vi "Max_Min_Delta.vi"() -> ()   [LabVIEW 2014]
panel:
  in  "OK Button 2":bool
  out "Delta":dbl
  out "Min":dbl
  out "Max":dbl
  in  "OK Button":bool
  in  "stop":bool
  out "Waveform Chart":dbl(graph)
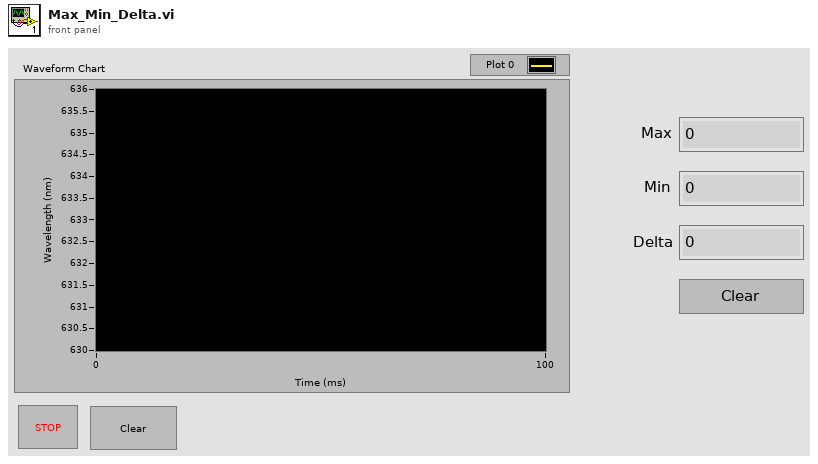
[diagram p1: front panel]
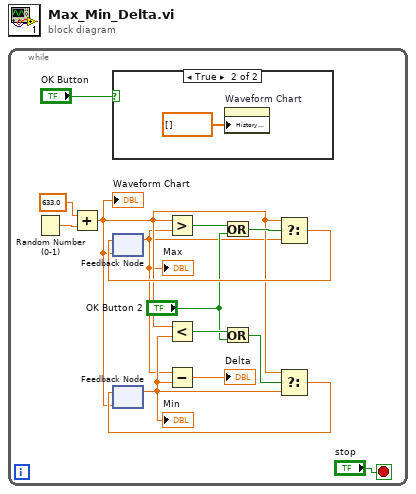
[diagram p0: block diagram]
diagram:
  n1 = while {
    stop <- "stop" stop-if-true
    n2 = Random Number (0-1)() -> (number: 0 to 1=w13:dbl)
    n3 = Add(x=633.0, y=w13) -> (x+y=w4:dbl)
    "Waveform Chart" <- w4
    n4 = case shown="True" "OK Button" {
      frame False {
      }
      frame True {
        n5 = property on="Waveform Chart" class="WFChart (strict)"("History Data"=dbl[] []) -> ()  [unwired: 2 in, 2 out]
      }
    }
    n6 = feedback #1(w4) -> (w1:dbl)
    "Max" <- w1
    n7 = feedback #2(w4) -> (w2:dbl)
    "Min" <- w2
    n8 = Greater?(x=w4, y=w1) -> (0:w11:bool)
    n9 = Less?(x=w4, y=w2) -> (x < y?=w8:bool)
    n10 = Subtract(x=w1, y=w2) -> (x-y=→"Delta":dbl)
    n11 = Or(x=w11, y="OK Button 2") -> (x .or. y?=w10:bool)
    n12 = Or(x=w8, y="OK Button 2") -> (x .or. y?=w7:bool)
    n13 = Select(t=w4, s=w10, f=w1) -> (s? t:f=w9:dbl)
    n14 = feedback-in #1(w9) -> ()
    n15 = Select(t=w4, s=w7, f=w2) -> (s? t:f=w6:dbl)
    n16 = feedback-in #2(w6) -> ()
  }
